vi "Add_Row_Times.vi"(3 "Start Index":i32, 5 "Table in":T1[](array[typedef]) {"Row Duration (mins)" format="%#.1f"; "Row No" min=0; "Trace Gas Concentration (%)" min=0.0 format="%#.2f"; "Emission Rate (l/min)" format="%#.2f"; "Tunnel Speed" format="%#.2f"; "Start X" format="%#.2f"; "Start Y" format="%#.2f"; "Start Z" format="%#.2f"; "End X" format="%#.2f"; "End Y" format="%#.2f"; "End Z" format="%#.2f"; "Averaging time (min)" min=0.0 format="%#.1f"}) -> (2 "Table Out":T1[](array[typedef]) {"Row Duration (mins)" format="%#.1f"; "Row No" min=0; "Trace Gas Concentration (%)" min=0.0 format="%#.2f"; "Emission Rate (l/min)" format="%#.2f"; "Tunnel Speed" format="%#.2f"; "Start X" format="%#.2f"; "Start Y" format="%#.2f"; "Start Z" format="%#.2f"; "End X" format="%#.2f"; "End Y" format="%#.2f"; "End Z" format="%#.2f"; "Averaging time (min)" min=0.0 format="%#.1f"})   [LabVIEW 2010]
uses:
  Traverse_cluster.ctl
  Spacing.ctl
  Controls/Multi_run_mode.ctl
  Controls/Overhead.ctl
panel:
  # "X           Y            Z"
  # "Start"
  # "End"
  # "X           Y            Z"
  # "Start"
  # "End"
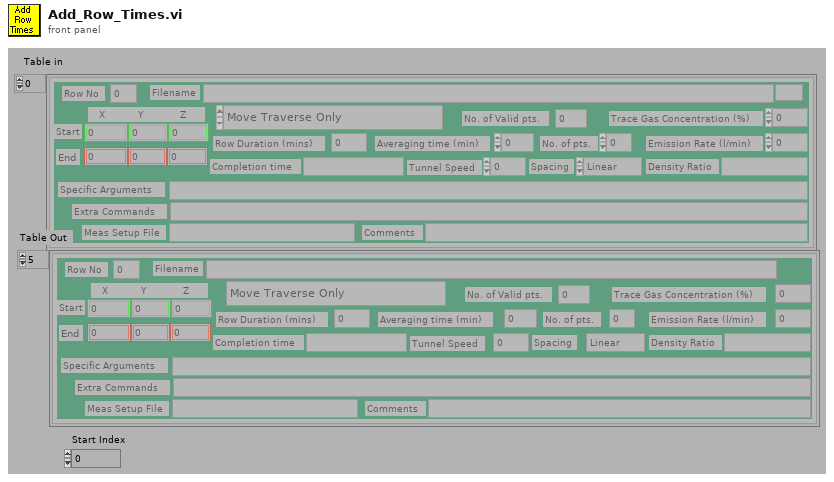
[diagram p1: front panel]
types:
  T1 = typedef "Traverse_cluster.ctl" = cluster{"Start X":dbl, "Start Y":dbl, "Start Z":dbl, "End X":dbl, "End Y":dbl, "End Z":dbl, "No. of pts.":i32, "Spacing":T2, "Filename":path, "Tunnel Speed":dbl, "Averaging time (min)":dbl, "Extra Commands":string, "Specific Arguments":string, "Emission Rate (l/min)":dbl, "Trace Gas Concentration (%)":dbl, "Density Ratio":string, "Comments":string, "Row No":i32, "Row Type Selector":T3, "Completion time":string, "Row Duration (mins)":dbl, "No. of Valid pts.":i32, "Meas Setup File":string}
  T2 = typedef "Spacing.ctl" = enum16{"Linear", "Log", "Gauss", "Specified", "N/A"}
  T3 = typedef "Multi_run_mode.ctl" = enum16{"Move Traverse Only", "Set Tunnel Speed Only", "Set Source Only", "Set Measurement Conditions", "Single Measurement", "Vertical Profile", "Lateral Profile", "Longitudinal Profile", "Explore Volume", "Multi-Axis Profile", "Auto Calibrate", "Meas Fast FID Bkgnd", "Check Beam Power", "Scanning Valve Measurement", "Run VI Named:", "Set ADAM Ch", "Wait (minutes)", "Send Message", "Synchronize With:", "Fall Back to this Row", "Turn Off Row Repeating", "Blank Row"}
  T4 = typedef "Overhead.ctl" = enum16{"Update total times", "Read Current Overhead", "Re Scale totals to 3 hrs", "Initialise totals to 3hr"}
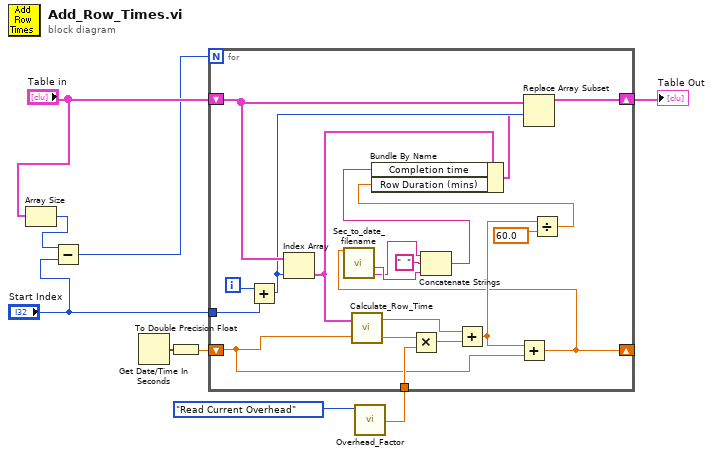
[diagram p0: block diagram]
diagram:
  n1 = Array Size(array="Table in") -> (size(s)=w7:i32)
  n2 = Subtract(x=w7, y="Start Index") -> (x-y=w5:i32)
  n3 = Get Date/Time In Seconds() -> (seconds since 1Jan1904=w1:timestamp)
  n4 = To Double Precision Float(number=w1) -> (double precision float=w4:dbl)
  n5 = call "Overhead_Factor.vi"("Mode"=Overhead."Read Current Overhead") -> ("Current Overhead Factor"=w2:dbl)  [unwired: 3 in]
  n6 = for {
    N: w5 -> [_]
    tunnel: "Start Index" -> [w28]
    shift-right: [w25] -> w9
    shift-left: "Table in" -> [w27]
    shift-right: [w12] -> _
    shift-left: w4 -> [w17]
    tunnel: w2 -> [w23]
    i -> [w29]
    n7 = Add(x=w29, y=w28) -> (x+y=w26:i32)
    n8 = Index Array(array=w27, index=w26) -> (element=w22:T1)
    n9 = call "Calculate_Row_Time.vi"("Row Start Time (Sec Since 1904)"=w17, "Multi Run Row"=w22) -> ("Scalable Time (Sec)"=w24:dbl, "Fixed Time (Sec)"=w20:dbl)
    n10 = Multiply(x=w24, y=w23) -> (x*y=w21:dbl)
    n11 = Add(x=w20, y=w21) -> (x+y=w13:dbl)
    n12 = Add(x=w13, y=w17) -> (x+y=w12:dbl)
    n13 = call "Sec_to_date_filename.vi"("seconds"=w12) -> ("Day"=w11:string, "Time"=w10:string)  [unwired: 2 out]
    n14 = Concatenate Strings(w10, "  " ("Substring"), w11) -> (w14:string)
    n15 = Divide(x=w13, y=60.0) -> (x/y=w18:dbl)
    n16 = Bundle By Name(cluster=w22, "Completion time"=w14, "Row Duration (mins)"=w18) -> (w16:T1)
    n17 = Replace Array Subset(array=w27, new element=w16, index=w26) -> (w25:T1[])
  }
  "Table Out" <- w9
